vi "PRL Check for bad dt.vi"(11 "Timestamp":timestamp[](array[timestamp])) -> (3 "Bad dt":bool)   [LabVIEW 2013, in "PMU Recorder Light.lvlib"]
uses:
  PMU Recorder Light.lvlib
  Setting Choice.ctl
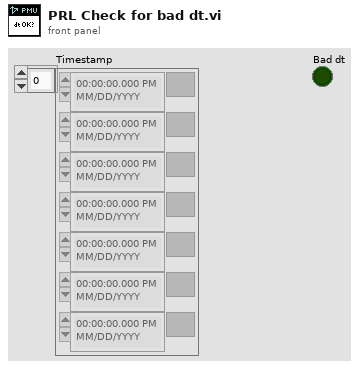
[diagram p1: front panel]
types:
  T1 = typedef "PMU Recorder Light.lvlib/Setting Choice.ctl" = enum16{"Analog Data Points Allowed Equals", "Complex Data Points Allowed Equals", "Seconds Before Reset After Wait for Config Fails", "Number of Live Buffer in Access Buffer ", "Number of Connection Attempts", "Live Data Buffer Size", "dt Tolerance", "Data Rate History", "ALL"}
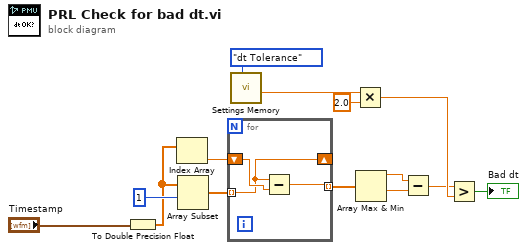
[diagram p0: block diagram]
diagram:
  n1 = To Double Precision Float(number="Timestamp") -> (double precision float=w5:dbl[])
  n2 = Index Array(array=w5) -> (element=w4:dbl)  [unwired: 1 in]
  n3 = Array Subset(array=w5, index=1) -> (w7:dbl[])  [unwired: 1 in]
  n4 = for {
    shift-right: [w15] -> _
    shift-left: w4 -> [w17]
    tunnel: w7 -> [w15] mode=indexing
    tunnel: [w16] -> w8 mode=indexing
    n5 = Subtract(x=w15, y=w17) -> (x-y=w16:dbl)
  }
  n6 = call "Settings Memory.vi"("Setting Choice"=Setting_Choice."dt Tolerance") -> ("PRL dt Tolerance"=w1:dbl)  [unwired: 8 in, 2 out]
  n7 = Multiply(x=w1, y=2.0) -> (x*y=w13:dbl)
  n8 = Array Max & Min(array=w8) -> (max value=w9:dbl, min value=w11:dbl)  [unwired: 2 out]
  n9 = Subtract(x=w9, y=w11) -> (x-y=w12:dbl)
  n10 = Greater?(x=w12, y=w13) -> (0:→"Bad dt":bool)
